vi "program seq..vi"(6 "IOList":T3, 7 "Cluster data":T5, 11 "Filepath":path=path "E:/My Project/2018-2019/Under development/Minda Ind. Switch -ID 144-145/Project/data/trail pro -12.txt") -> (0 "Error Out":errorcluster)   [LabVIEW 2015]
uses:
  Control PB/Active.ctl
  Control PB/deactive.ctl
  Control PB/output control.ctl
  Control PB/input control.ctl
  Control PB/timer.ctl
  Control PB/Remove list.ctl
  Control Button/Exit.ctl
  Control PB/Add_s.ctl
  Control PB/Delete_.ctl
  Control Button/Save.ctl
  Control PB/motor.ctl
  Control PB/Camera.ctl
  Control PB/Barcode.ctl
  Galobal variable_TI.vi
panel:
  out "Step List 4":string[](array[string])
  out "Step List 3":string[](array[string])
  in  "Barcode":T1
  in  "Camera":T2
  out "x <= y?":bool
  out "Cancel":bool
  out "Step List 2":string[](array[string])
  out "Pokayoka Result":cluster{"Sensor Name":string, "Boolean":bool}[](array[cluster])
  in  "Feed Back Channel":i32[](listbox)=[0]
  out "Input":bool[](array[boolean])
  out "Feature List (Out) 2":T4(array[cluster])
  out "error out 2":errorcluster
  in  "Control":bool
  out "Station No":string
  out "Model Name":string
  out "Model":string
  in  "Motor":T6
  in  "Feature List":i32(listbox) caption="Steps List"
  in  "Deletefeature list":T7
  in  "Add feature list":T8
  in  "Deactive":T9
  in  "Active":T10
  in  "Program step":i32(listbox)
  in  "Remove Step":T11
  in  "Wait Time":u32=100 caption="Timer(ms)" max=600000 step=1
  in  "Timer":T12
  in  "Save":T13
  in  "stop":T14
  in  "op Add":T15
  in  "Input Add":T16
  out "Step List":string[](array[string])
  out "output cluster":T17
  in  "Analog":bool
  in  "Analog Input":i32[](listbox)=[0]
  in  "Control Channel":i32[](listbox)=[7]
  in  "Steps":T18(array[cluster])
  in  "Program mode":string="Data"
  out "error out":errorcluster
  out "Feature List (Out)":T19(array[cluster])
  # "Program Sequence Window"
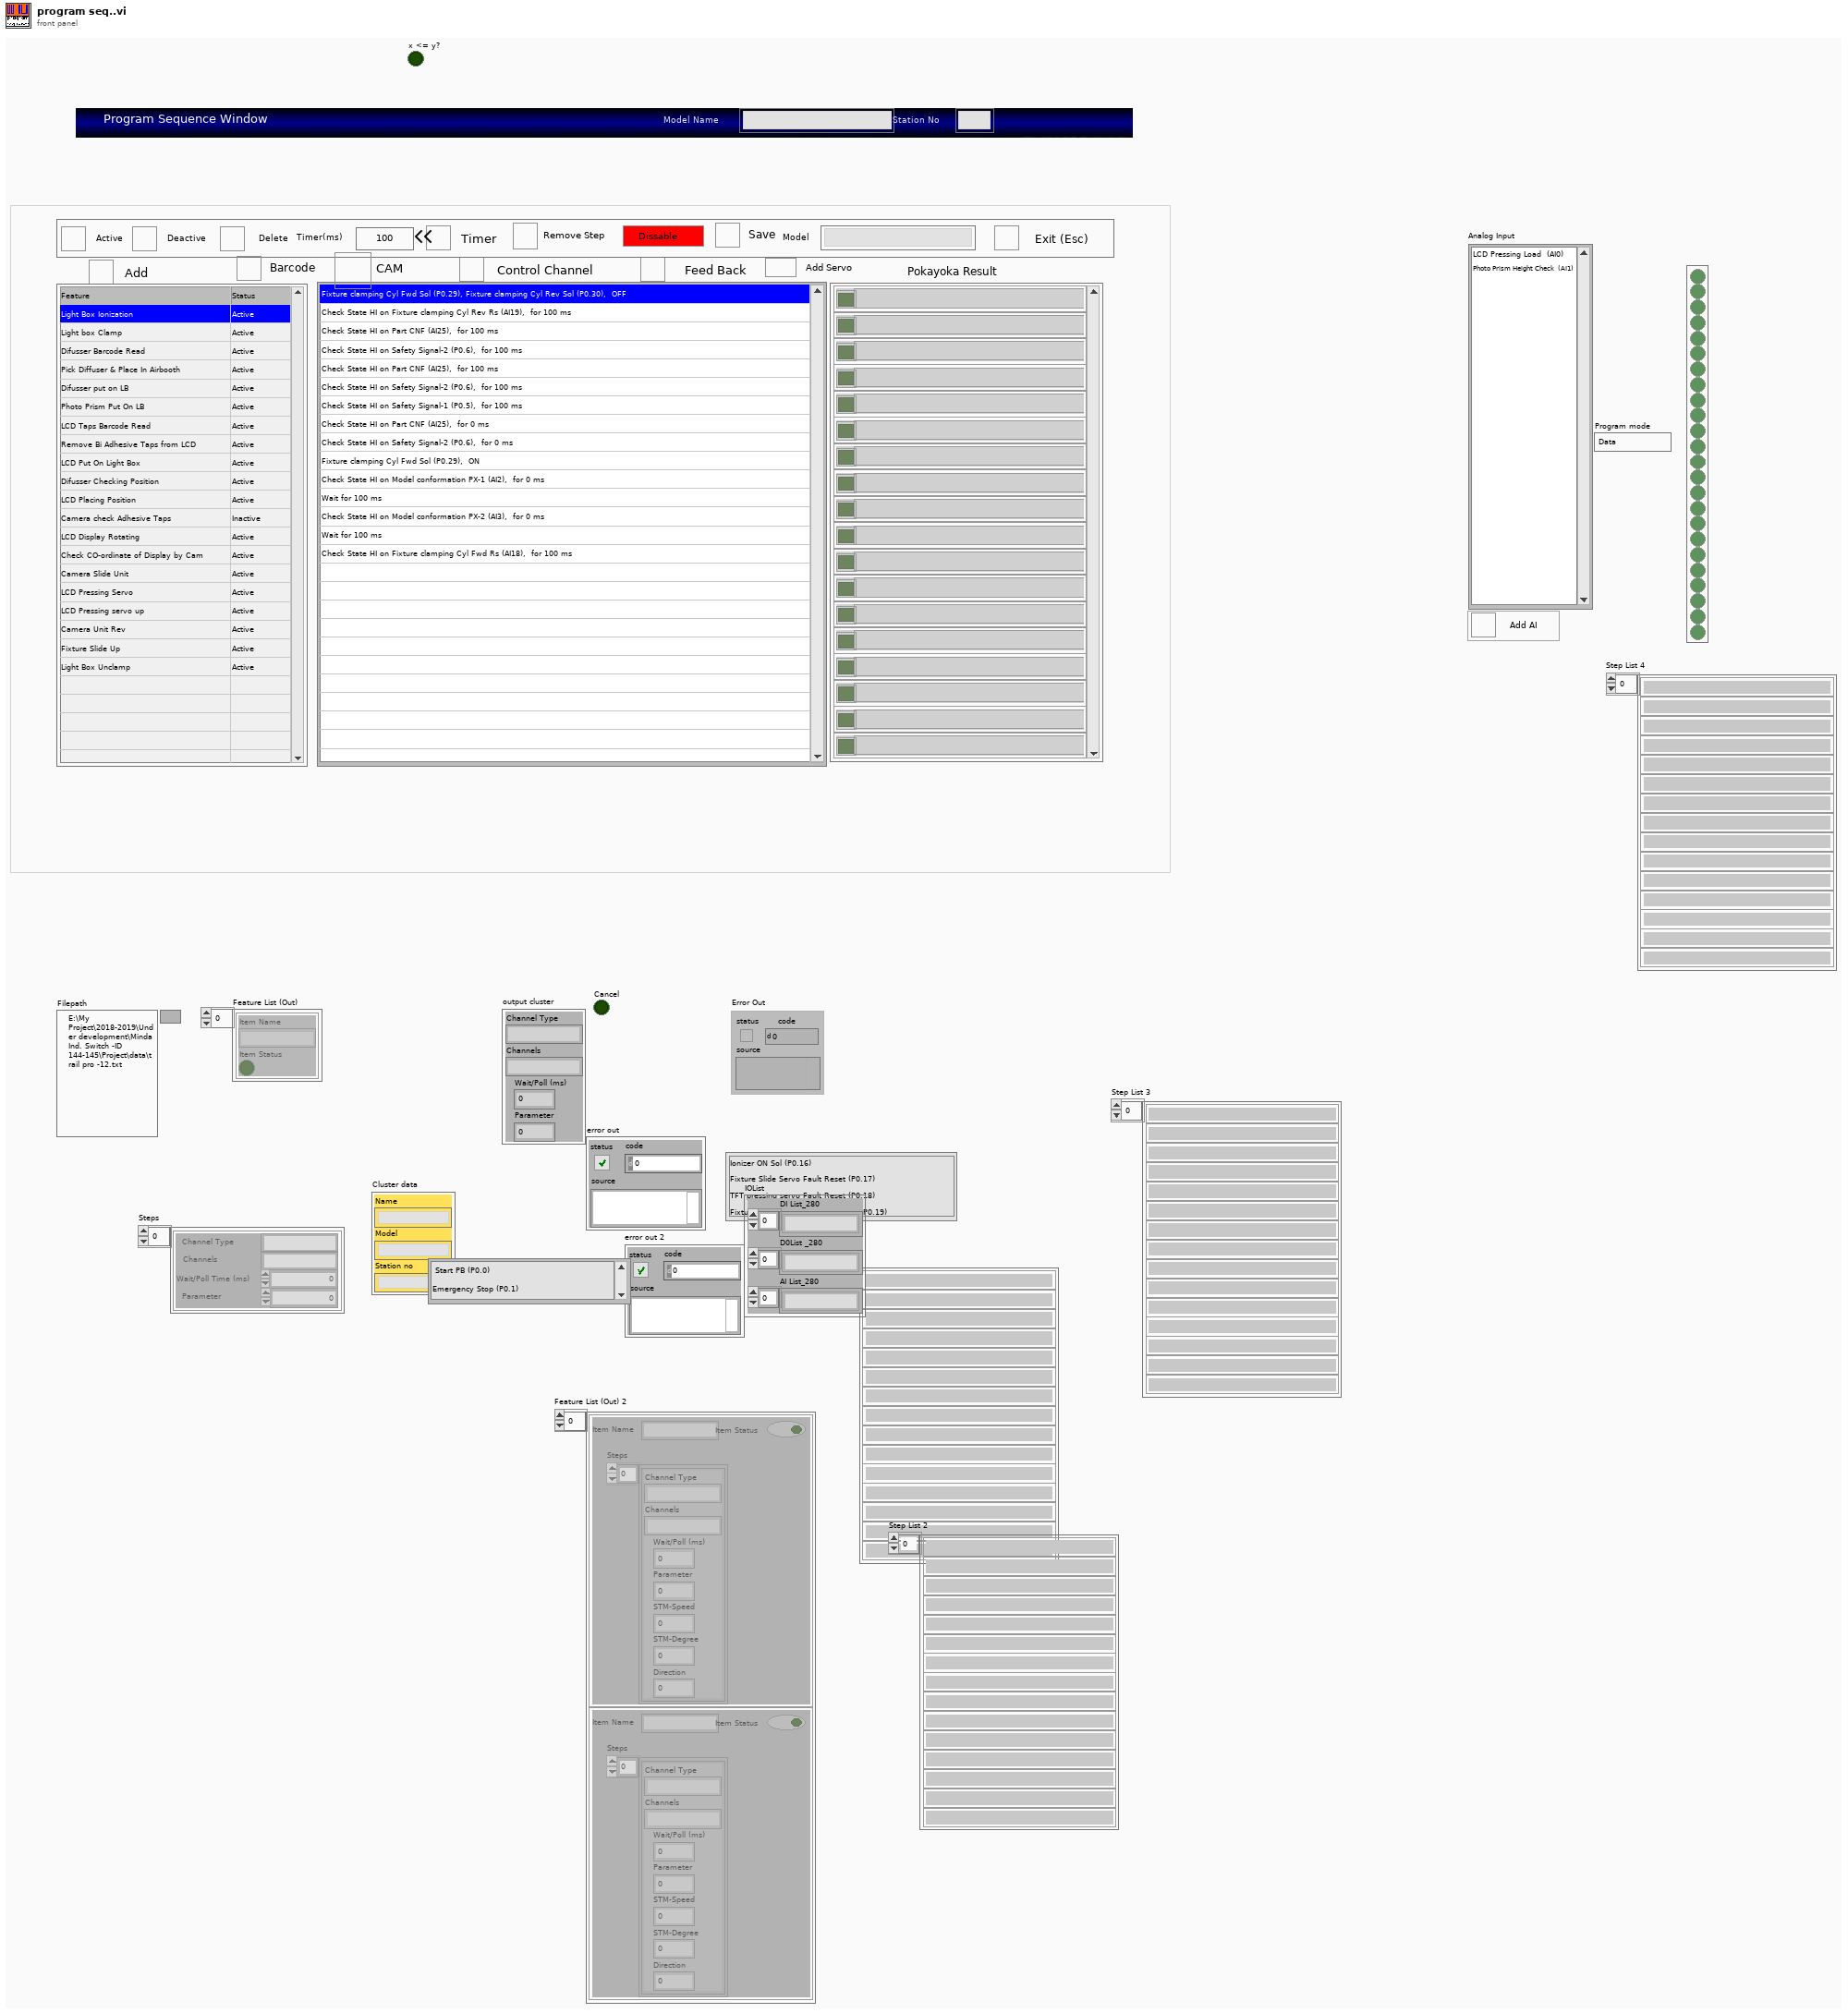
[diagram p1: front panel]
types:
  T1 = typedef "Barcode.ctl" = bool
  T2 = typedef "Camera.ctl" = bool
  T3 = cluster{"DI List_280":string[], "D0List _280":string[], "AI List_280":string[]}
  T4 = cluster{"Item Name":string, "Item Status":bool, "Steps":cluster{"Channel Type":string, "Channels":string, "Wait/Poll (ms)":u32, "Parameter":u8, "STM-Speed":i32, "STM-Degree":u32, "Direction":u8}[]}[]
  T5 = cluster{"Name":string, "Model":string, "Station no":string}
  T6 = typedef "motor.ctl" = bool
  T7 = typedef "Delete_.ctl" = bool
  T8 = typedef "Add_s.ctl" = bool
  T9 = typedef "deactive.ctl" = bool
  T10 = typedef "Active.ctl" = bool
  T11 = typedef "Remove list.ctl" = bool
  T12 = typedef "timer.ctl" = bool
  T13 = typedef "Save.ctl" = bool
  T14 = typedef "Exit.ctl" = bool
  T15 = typedef "output control.ctl" = bool
  T16 = typedef "input control.ctl" = bool
  T17 = cluster{"Channel Type":string, "Channels":string, "Wait/Poll (ms)":u32, "Parameter":u8}
  T18 = cluster{"Channel Type":string, "Channels":string, "Wait/Poll Time (ms)":u32, "Parameter":u8}[]
  T19 = cluster{"Item Name":string, "Item Status":bool}[]
  T20 = cluster{"Channel Type":string, "Channels":string, "Wait/Poll (ms)":u32, "Parameter":u8, "STM-Speed":i32, "STM-Degree":i32, "Direction":u8}
  T21 = cluster{"Item Name":string, "Item Status":bool, "Steps":cluster{"Channel Type":string, "Channels":string, "Wait/Poll (ms)":u32, "Parameter":u8, "STM-Speed":i32, "STM-Degree":u32, "Direction":u8}[]}
  T22 = cluster{"Channel Type":string, "Channels":string, "Wait/Poll (ms)":u32, "Parameter":u8, "STM-Speed":i32, "STM-Degree":u32, "Direction":u8}[]
  T23 = cluster{"Item Name":string, "Active":T10, "Steps":cluster{"Channel Type":string, "Channels":string, "Wait/Poll (ms)":u32, "Parameter":u8, "STM-Speed":i32, "STM-Degree":u32, "Direction":u8}[]}
  T24 = cluster{"Channel Type":string, "Channels":string, "Wait/Poll (ms)":u32, "Parameter":u8, "STM-Speed":i32, "STM-Degree":i32, "Direction":u8}[]
  T25 = cluster{"Feature name ":string, bool, cluster{"Channel Type":string, "Channels":string, "Wait/Poll (ms)":u32, "Parameter":u8, "STM-Speed":i32, "STM-Degree":i32, "Direction":u8}[]}
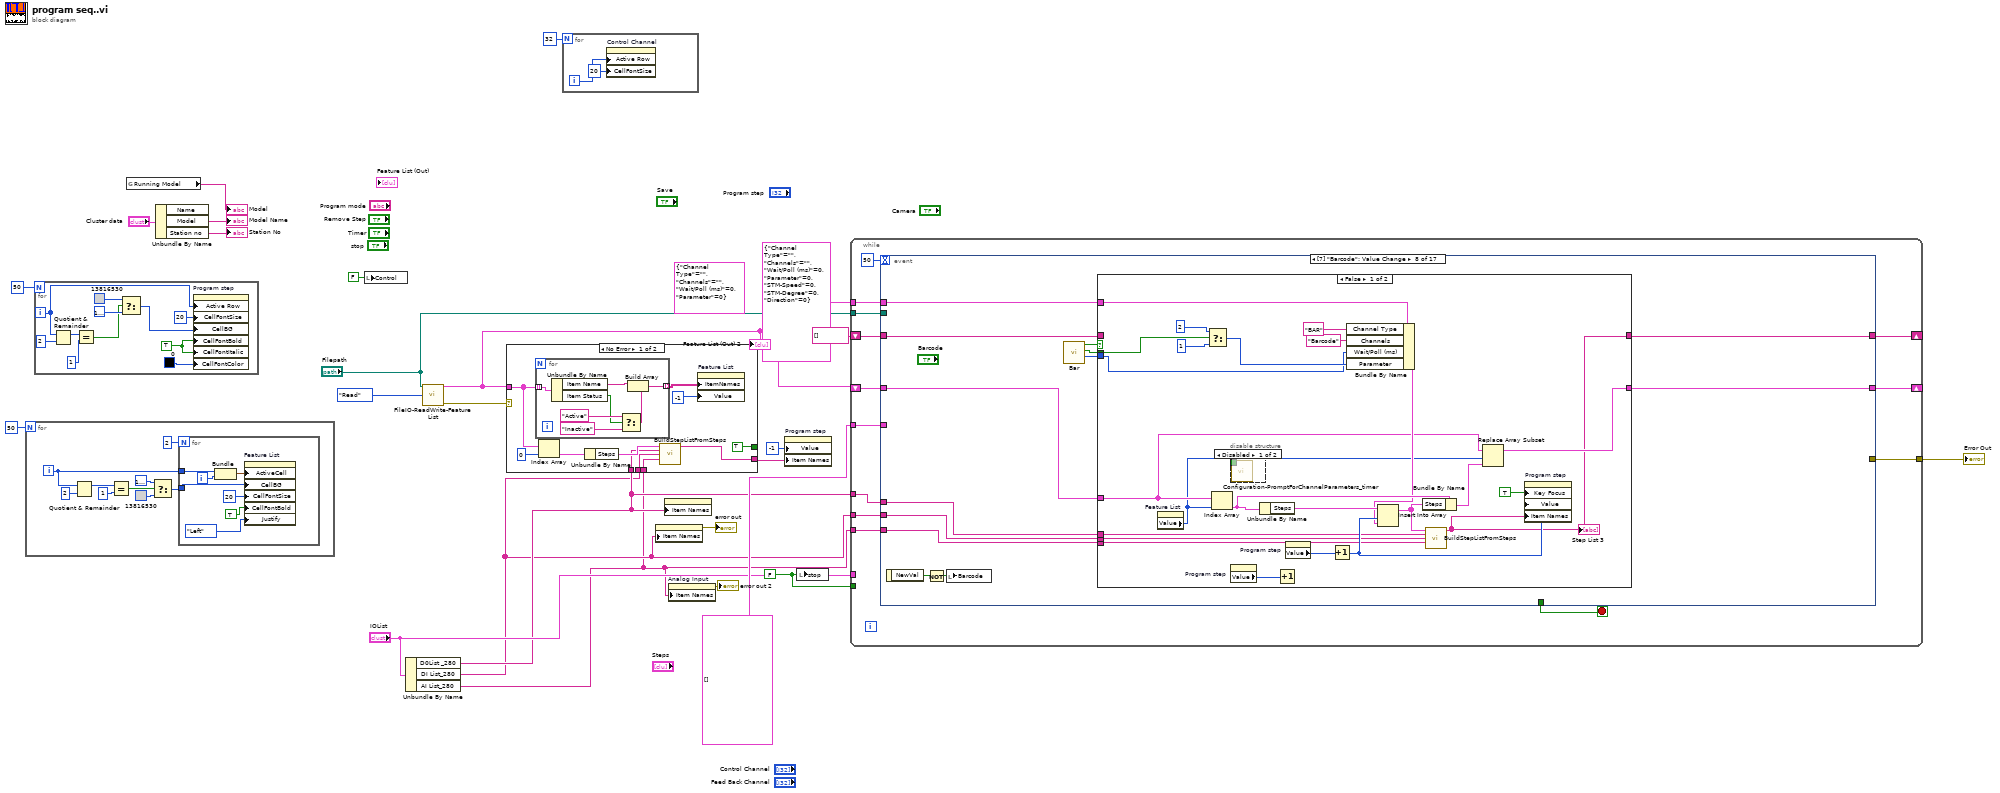
[diagram p0: block diagram]
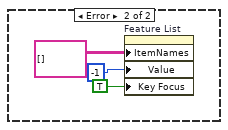
[diagram p2: hidden frame]
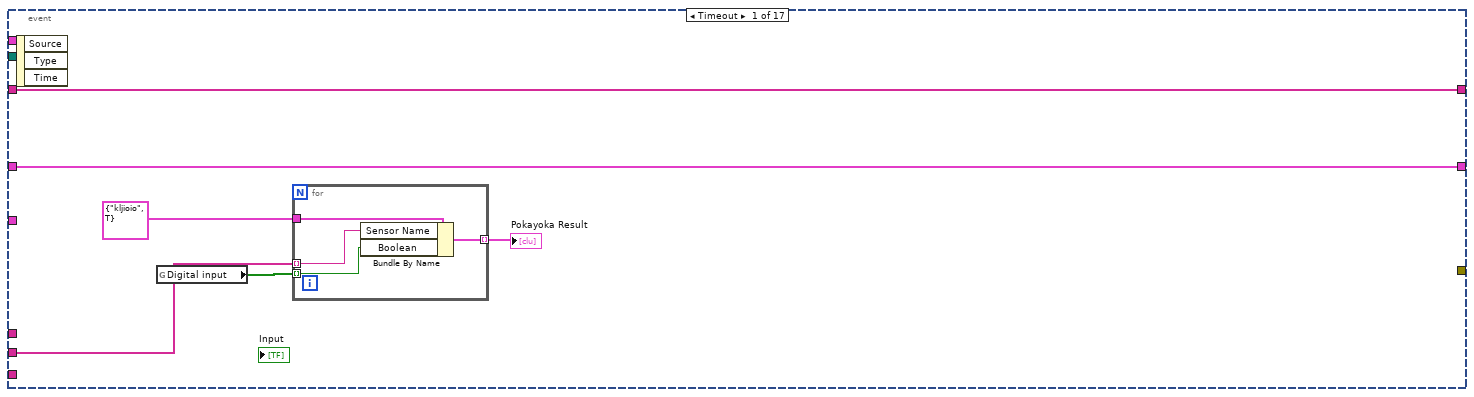
[diagram p3: hidden frame]
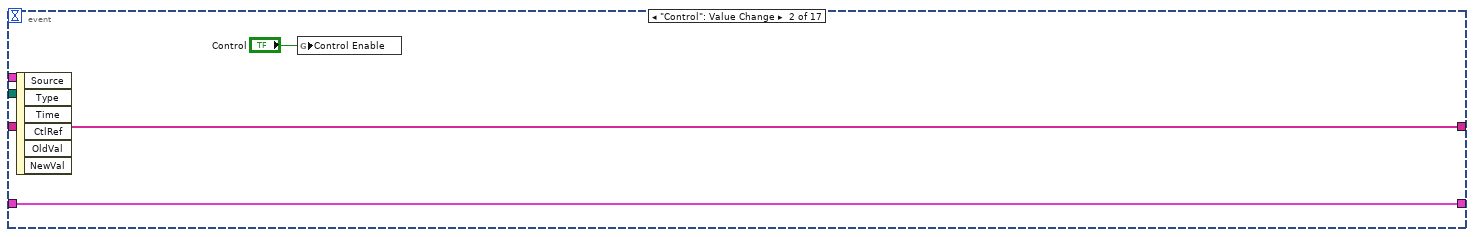
[diagram p4: hidden frame]
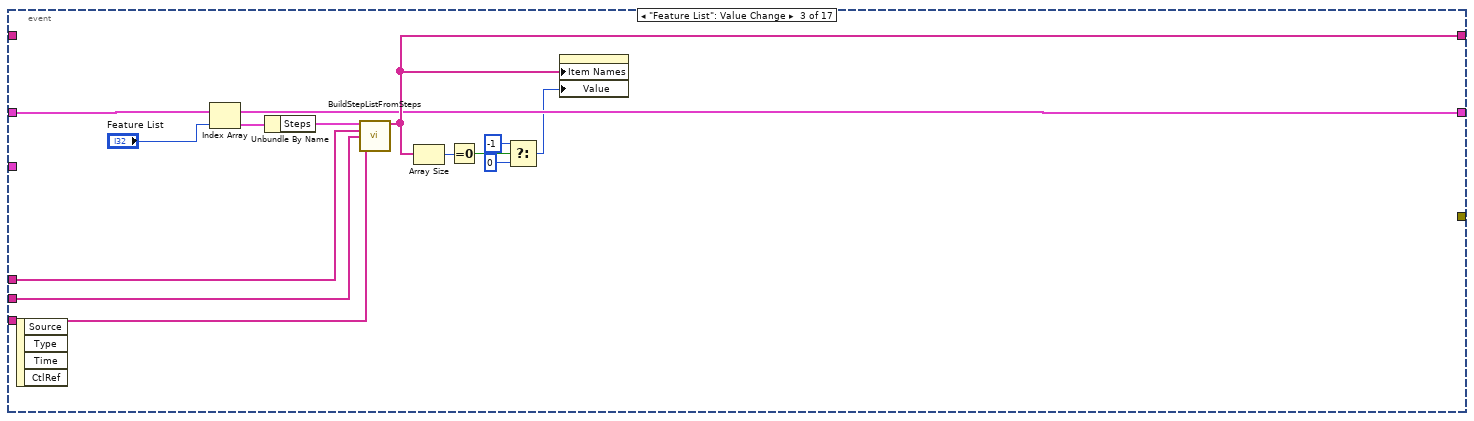
[diagram p5: hidden frame]
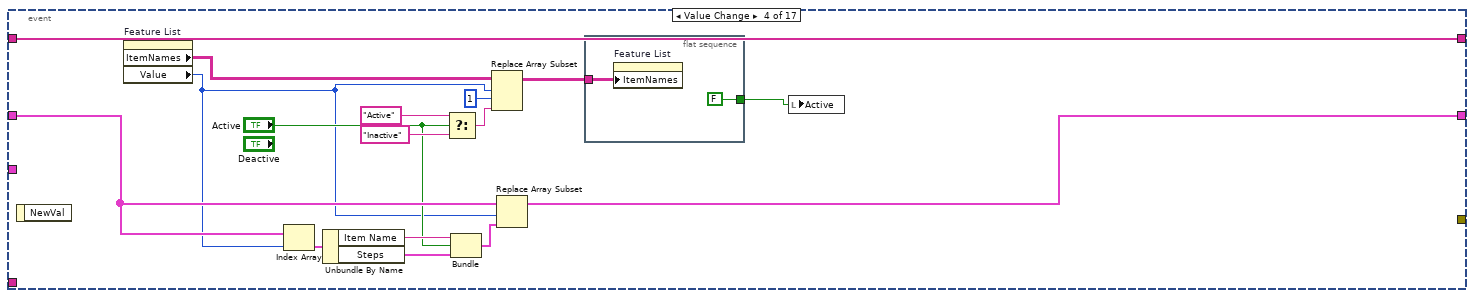
[diagram p6: hidden frame]
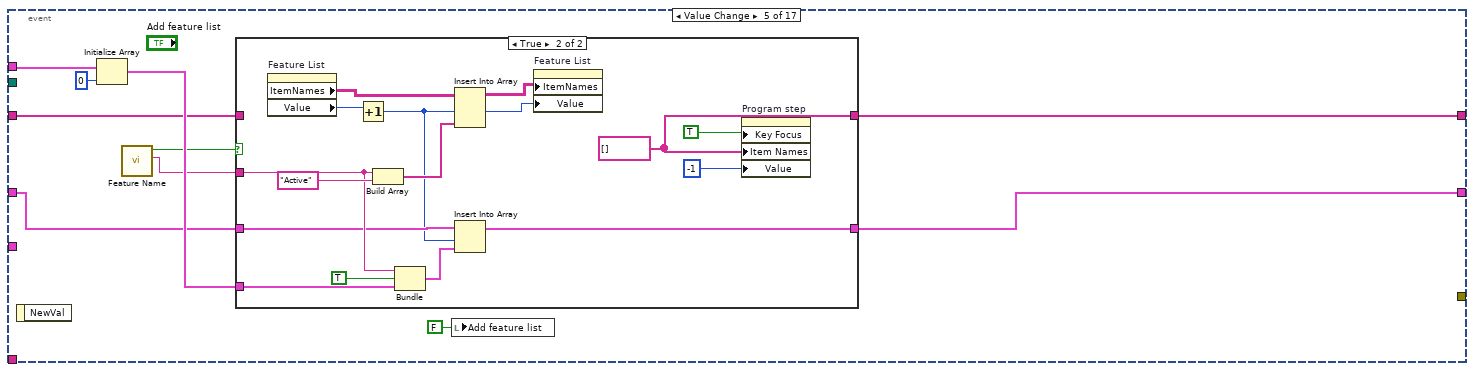
[diagram p7: hidden frame]
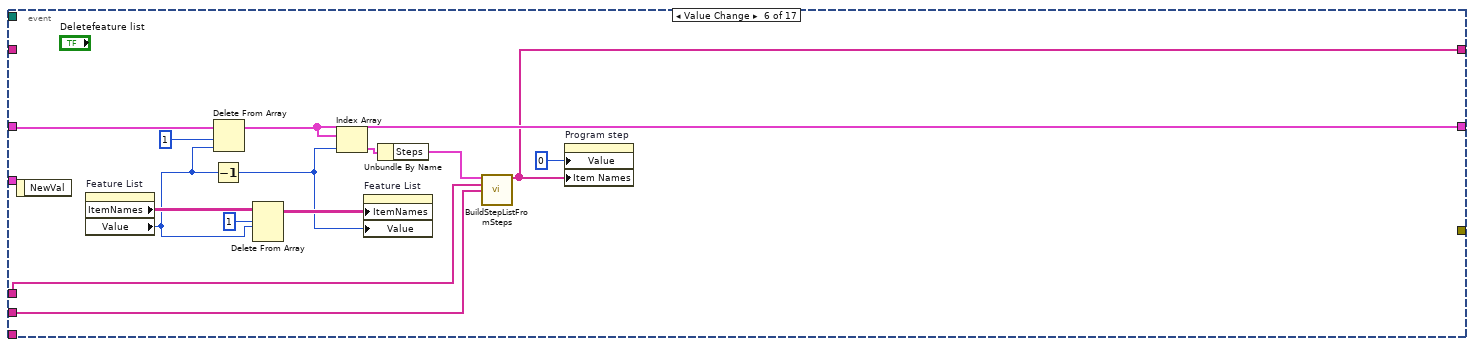
[diagram p9: hidden frame]
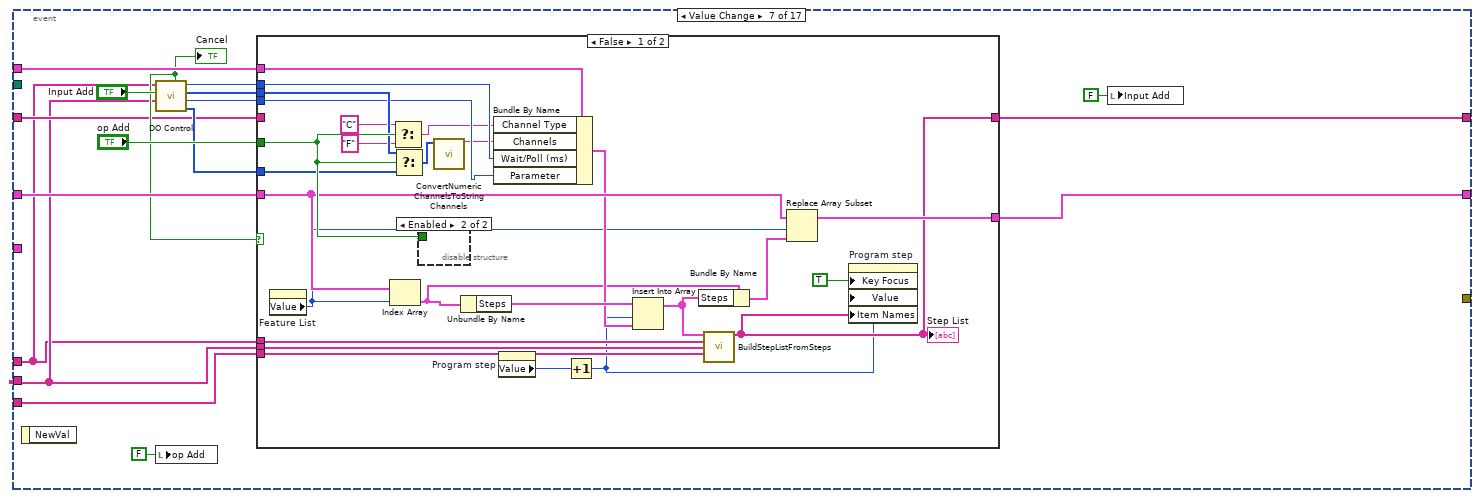
[diagram p10: hidden frame]
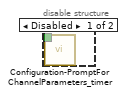
[diagram p11: hidden frame]
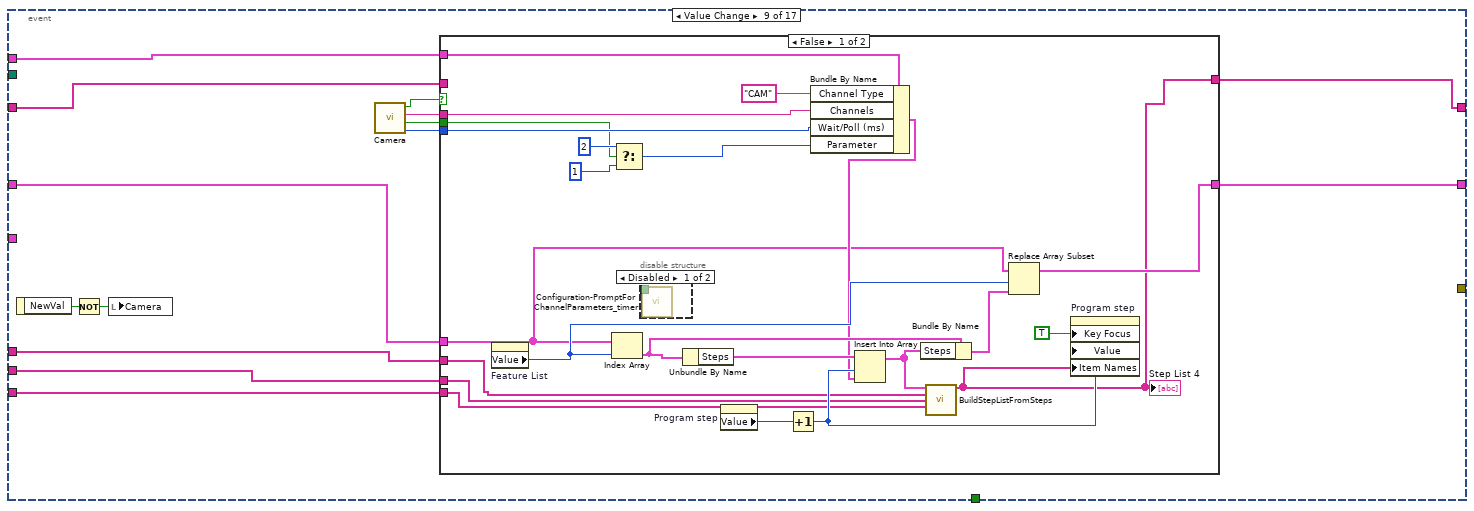
[diagram p15: hidden frame]
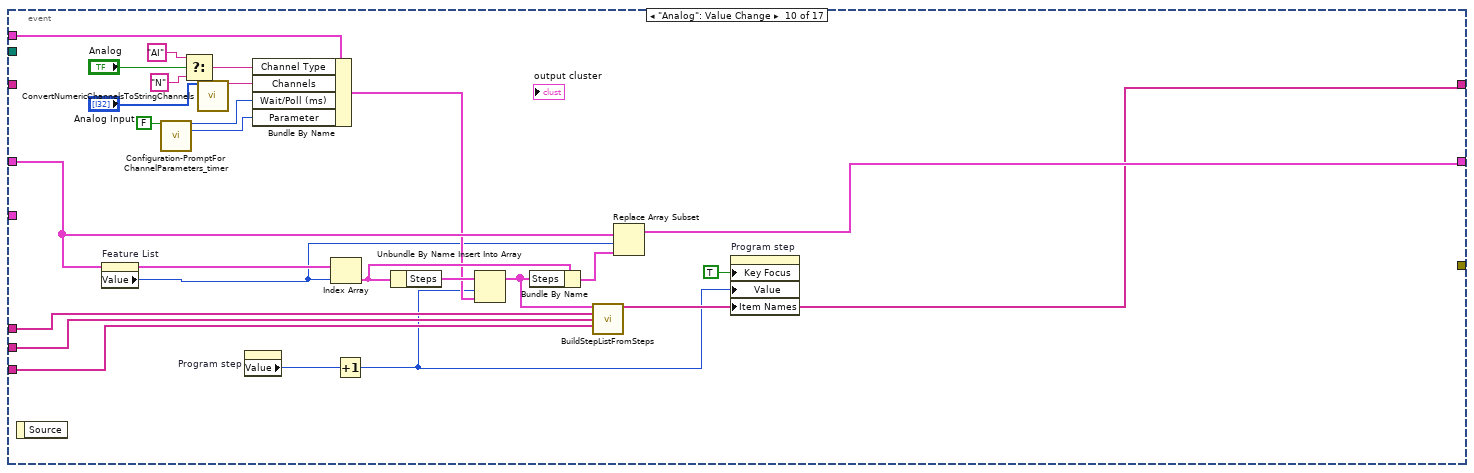
[diagram p18: hidden frame]
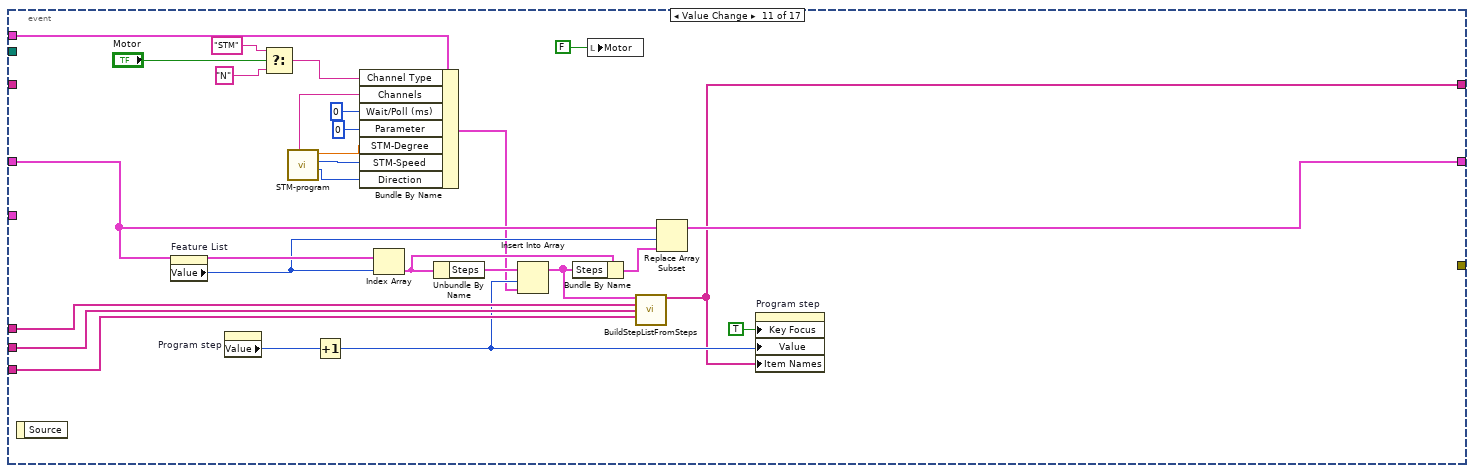
[diagram p19: hidden frame]
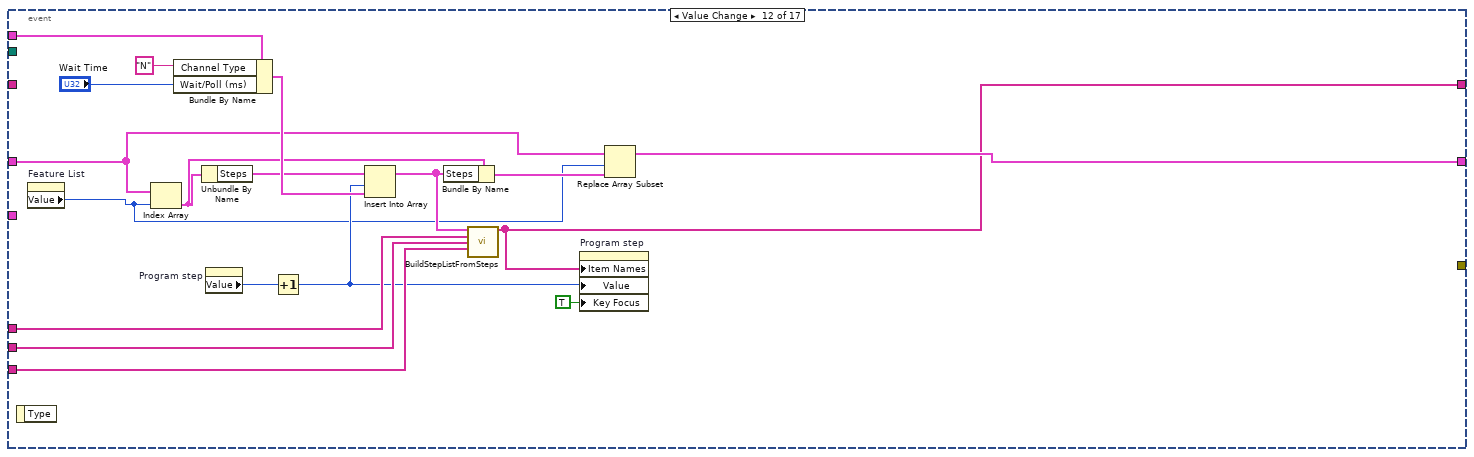
[diagram p20: hidden frame]
diagram:
  w9 = FALSE ("stop")
  (unwired) T17 {"Channel Type"="", "Channels"="", "Wait/Poll (ms)"=0, "Parameter"=0} ("Step")
  n1 = for {
    N: 50 -> [_]
    i -> [w33]
    n2 = Quotient & Remainder(x=w33, y=2) -> (x-y*floor(x/y)=w31:i32)  [unwired: 1 out]
    n3 = Equal?(x=w31, y=1) -> (x = y?=w29:bool)
    n4 = Select(t=u32 16777225 ("Color Box"), s=w29, f=u32 13816530 ("Color Box")) -> (s? t:f=w26:u32)
    n5 = for {
      N: 2 -> [_]
      tunnel: w33 -> [w41]
      tunnel: w26 -> [w38]
      i -> [w40]
      n6 = Bundle(w41, w40) -> (w39:cluster{i32, i32})  [unwired: 1 in]
      n7 = property on="Feature List" class="MCListbox (strict)"("ActiveCell"=w39, "CellBG"=w38, "CellFontSize"=u32 20 ("Active Cell:Cell Font:Size"), "CellFontBold"=TRUE ("Active Cell:Cell Font:Bold"), "Justify"=enum16{"Left", "Center", "Right"}."Left" ("Active Cell:Cell Justification")) -> ()  [unwired: 2 in, 2 out]
    }
  }
  n8 = for {
    N: 50 -> [_]
    i -> [w46]
    w43 = TRUE
    n9 = Quotient & Remainder(x=w46, y=2) -> (x-y*floor(x/y)=w49:i32)  [unwired: 1 out]
    n10 = Equal?(x=w49, y=1) -> (x = y?=w47:bool)
    n11 = Select(t=u32 13816530 ("Color Box"), s=w47, f=u32 16777226 ("Color Box")) -> (s? t:f=w44:u32)
    n12 = property on="Program step" class="LstBox (strict)"("Active Row"=w46, "CellFontSize"=u32 20 ("Active Row:Cell Font:Size"), "CellBG"=w44, "CellFontBold"=w43, "CellFontItalic"=w43, "CellFontColor"=u32 0 ("Color Box")) -> ()  [unwired: 2 in, 2 out]
  }
  n13 = global read "Galobal variable_TI.vi" "Running Model"() -> (→"Model":string)
  n14 = Unbundle By Name("Cluster data") -> ("Model"=→"Model Name":string, "Station no"=→"Station No":string)  [unwired: 1 out]
  n15 = local write "Control"(FALSE ("Control")) -> ()
  n16 = Unbundle By Name("IOList") -> ("D0List _280"=w5:string[], "DI List_280"=w4:string[], "AI List_280"=w3:string[])
  n17 = call "FileIO-ReadWrite-FeatureList.vi"("Filepath"="Filepath", "Read/Write"=enum16{"Read", "Write"}."Read") -> ("Feature List (Out)"=w16:T4, "Error Out"=w20:errorcluster)  [unwired: 12 in]
  "Feature List (Out) 2" <- w16
  n18 = case shown="No Error" w20 {
    tunnel: w16 -> [w63 _]
    tunnel: w5 -> [w59 _]
    tunnel: w4 -> [w58 _]
    tunnel: w3 -> [w57 _]
    tunnel: [w56 _] -> w19
    tunnel: [TRUE ("Key Focus") _] -> _
    frame No Error {
      n19 = for {
        tunnel: w63 -> [w70] mode=indexing
        tunnel: [w64] -> w54 mode=indexing
        n20 = Unbundle By Name(w70) -> ("Item Name"=w66:string, "Item Status"=w67:bool)
        n21 = Select(t="Active", s=w67, f="Inactive") -> (s? t:f=w65:string)
        n22 = Build Array(w66, w65) -> (w64:string[])
      }
      n23 = Index Array(array=w63, index=0) -> (element=w61:T21)
      n24 = Unbundle By Name(w61) -> ("Steps"=w60:T22)
      n25 = call "BuildStepListFromSteps.vi"("Steps"=w60, "Control Channels"=w59, "Feedback Channels"=w58, "AI"=w57) -> ("Step List"=w56:string[])  [unwired: 11 in]
      n26 = property on="Feature List" class="MCListbox (strict)"("ItemNames"=w54, "Value"=-1 ("Feautre list")) -> ()  [unwired: 2 in, 2 out]
    }
    frame Error {
      n27 = property on="Feature List" class="MCListbox (strict)"("ItemNames"=string[][] [] ("Item Names"), "Value"=-1 ("Feautre list"), "Key Focus"=TRUE) -> ()  [unwired: 2 in, 2 out]
    }
  }
  n28 = for {
    N: 32 -> [_]
    i -> [w75]
    n29 = property on="Control Channel" class="LstBox (strict)"("Active Row"=w75, "CellFontSize"=u32 20 ("Active Row:Cell Font:Size")) -> ()  [unwired: 2 in, 2 out]
  }
  n30 = property on="Feed Back Channel" class="LstBox (strict)"("Item Names"=w4) -> (error out=→"error out":errorcluster)  [unwired: 2 in, 1 out]
  n31 = property on="Control Channel" class="LstBox (strict)"("Item Names"=w5) -> ()  [unwired: 2 in, 2 out]
  n32 = property on="Analog Input" class="LstBox (strict)"("Item Names"=w3) -> (error out=→"error out 2":errorcluster)  [unwired: 2 in, 1 out]
  n33 = property on="Program step" class="LstBox (strict)"("Value"=-1 ("Step feautre list"), "Item Names"=w19) -> ()  [unwired: 2 in, 2 out]
  n34 = local write "stop"(w9) -> ()
  n35 = while {
    shift-right: [w86] -> _
    shift-left: w16 -> [w77]
    tunnel: T20 {"Channel Type"="", "Channels"="", "Wait/Poll (ms)"=0, "Parameter"=0, "STM-Speed"=0, "STM-Degree"=0, "Direction"=0} ("Step") -> [w87]
    shift-right: [w85] -> _
    shift-left: string[] [] ("Step List") -> [w84]
    tunnel: w5 -> [w83]
    tunnel: w4 -> [w82]
    tunnel: [w81] -> w23
    tunnel: w3 -> [w80]
    tunnel: T4 [] ("Feature List (Out) 2") -> [w79]
    tunnel: "Filepath" -> [w78]
    tunnel: w9 -> [_]
    tunnel: "IOList" -> [_]
    stop <- w88 stop-if-true
    n36 = event shown="[7] \"Barcode\": Value Change" {
      selector: _ -> [_ _ _ _ _ _ _ _ _ _ _ _ _ _ _ _ _]
      dyn-events: _ -> [_ _ _ _ _ _ _ _ _ _ _ _ _ _ _ _ _]
      timeout: 50 -> [_ _ _ _ _ _ _ _ _ _ _ _ _ _ _ _ _]
      tunnel: [_ _ _ _ _ _ _ _ _ _ _ _ _ _ TRUE ("stop") _ TRUE ("Discard?")] -> w88
      tunnel: w77 -> [w94 w100 w105 w122 w139 w171 w187 w227 w269 w309 w339 w360 w382 w391 w451 w473 w550]
      tunnel: w87 -> [_ _ _ _ w142 _ w190 w232 w273 w316 w344 w369 _ _ _ w474 _]
      tunnel: [w94 w100 w105 w120 w138 w170 w188 w226 w268 w304 w331 w359 w381 w393 w451 w469 w550] -> w86
      tunnel: [w93 w101 w108 w119 w135 w165 w186 w225 w267 w303 w330 w356 w376 w408 w450 w468 w551] -> w85
      tunnel: w84 -> [w93 w101 _ w119 w134 _ w177 w220 w263 _ _ _ _ _ w450 w467 w551]
      tunnel: w83 -> [_ _ w107 _ _ w167 w175 w228 w270 w306 w336 w358 w378 w410 _ w470 _]
      tunnel: w82 -> [w92 _ w106 _ _ w166 w176 w229 w271 w307 w335 w357 w377 w409 _ w471 _]
      tunnel: [_ _ _ _ _ _ _ _ _ _ _ _ _ w401 _ _ _] -> w81
      tunnel: w80 -> [_ _ w104 _ _ _ w185 w230 w272 w308 w334 w355 _ w402 _ w472 _]
      tunnel: w79 -> [_ _ _ _ _ _ _ _ _ _ _ _ _ w407 _ _ _]
      tunnel: w78 -> [_ _ _ _ _ _ _ _ _ _ _ _ _ w392 _ _ _]
      event Timeout {
        n37 = event-data() -> ()  [unwired: 1 in, 3 out]
        n38 = global read "Galobal variable_TI.vi" "Digital input"() -> (w89:bool[])
        n39 = for {
          tunnel: w92 -> [w97] mode=indexing
          tunnel: cluster{"Sensor Name":string, "Boolean":bool} {"Sensor Name"="kljioio", "Boolean"=TRUE} ("Cluster") -> [w98]
          tunnel: [w96] -> w90 mode=indexing
          tunnel: w89 -> [w95] mode=indexing
          n40 = Bundle By Name(cluster=w98, "Sensor Name"=w97, "Boolean"=w95) -> (w96:cluster{"Sensor Name":string, "Boolean":bool})
        }
        "Pokayoka Result" <- w90
      }
      event "Control": Value Change {
        n41 = event-data() -> ()  [unwired: 1 in, 6 out]
        n42 = global write "Galobal variable_TI.vi" "Control Enable"("Control") -> ()
      }
      event "Feature List": Value Change {
        n43 = event-data() -> ()  [unwired: 1 in, 4 out]
        n44 = Index Array(array=w105, index="Feature List") -> (element=w114:T21)
        n45 = Unbundle By Name(w114) -> ("Steps"=w113:T22)
        n46 = call "BuildStepListFromSteps.vi"("Steps"=w113, "Control Channels"=w107, "Feedback Channels"=w106, "AI"=w104) -> ("Step List"=w108:string[])  [unwired: 11 in]
        n47 = Array Size(array=w108) -> (size(s)=w110:i32)
        n48 = Equal To 0?(x=w110) -> (x = 0?=w112:bool)
        n49 = Select(t=-1 ("Step List"), s=w112, f=0 ("Step List")) -> (s? t:f=w103:i32)
        n50 = property on="Program step" class="LstBox (strict)"("Item Names"=w108, "Value"=w103) -> ()  [unwired: 2 in, 2 out]
      }
      event Value Change {
        n51 = event-data() -> ()  [unwired: 1 in, 1 out]
        n52 = property on="Feature List" class="MCListbox (strict)"() -> ("ItemNames"=w118:string[][], "Value"=w116:i32)  [unwired: 2 in, 2 out]
        n53 = Index Array(array=w122, index=w116) -> (element=w128:T21)
        n54 = Unbundle By Name(w128) -> ("Item Name"=w129:string, "Steps"=w130:T22)
        n55 = Select(t="Active", s="Active", f="Inactive" ("element")) -> (s? t:f=w125:string)
        n56 = Bundle("Item Name"=w129, "Active"="Active", "Steps"=w130) -> (w127:T23)  [unwired: 1 in]
        n57 = Replace Array Subset(array=w118, new element=w125, index (row)=w116, index (col)=1 ("disabled index (col)")) -> (w117:string[][])
        n58 = Replace Array Subset(array=w122, new element=w127, index=w116) -> (w120:T4)
        n59 = flat-sequence {
          tunnel: w117 -> [w132]
          tunnel: [T10 FALSE ("Active")] -> w115
          frame #0 {
            n60 = property on="Feature List" class="MCListbox (strict)"("ItemNames"=w132) -> ()  [unwired: 2 in, 2 out]
          }
        }
        n61 = local write "Active"(w115) -> ()
      }
      event Value Change {
        n62 = event-data() -> ()  [unwired: 1 in, 1 out]
        n63 = Initialize Array(w142, 0 ("dimension size")) -> (w140:T24)
        n64 = call "Feature Name.vi"() -> ("Feature name"=w136:string, "Out"=w137:bool)  [unwired: 10 in]
        n65 = case shown="True" w137 {
          tunnel: w140 -> [_ w158]
          tunnel: w139 -> [w144 w153]
          tunnel: [w144 w155] -> w138
          tunnel: w136 -> [_ w154]
          tunnel: [w143 w151] -> w135
          tunnel: w134 -> [w143 _]
          frame False {
          }
          frame True {
            w151 = string[] [] ("Item Names")
            n66 = property on="Feature List" class="MCListbox (strict)"() -> ("ItemNames"=w148:string[][], "Value"=w145:i32)  [unwired: 2 in, 2 out]
            n67 = Increment(x=w145) -> (x+1=w146:i32)
            n68 = Build Array(w154, "Active") -> (w149:string[])
            n69 = Bundle("Feature name"=w154, TRUE, w158) -> (w156:T25)  [unwired: 1 in]
            n70 = Insert Into Array(array=w148, index (row)=w146, new element=w149) -> (w147:string[][])  [unwired: 1 in]
            n71 = Insert Into Array(array=w153, index=w146, new element=w156) -> (w155:T4)
            n72 = property on="Feature List" class="MCListbox (strict)"("ItemNames"=w147, "Value"=w146) -> ()  [unwired: 2 in, 2 out]
            n73 = property on="Program step" class="LstBox (strict)"("Key Focus"=TRUE, "Item Names"=w151, "Value"=-1 ("Step feautre list")) -> ()  [unwired: 2 in, 2 out]
          }
        }
        n74 = local write "Add feature list"(FALSE ("Add feature list")) -> ()
      }
      event Value Change {
        n75 = event-data() -> ()  [unwired: 1 in, 1 out]
        n76 = property on="Feature List" class="MCListbox (strict)"() -> ("ItemNames"=w163:string[][], "Value"=w162:i32)  [unwired: 2 in, 2 out]
        n77 = Decrement(x=w162) -> (x-1=w160:i32)
        n78 = Delete From Array(array=w171, length=1, index=w162) -> (array with subset deleted=w170:T4)  [unwired: 1 out]
        n79 = Delete From Array(array=w163, length=1, index (row)=w162) -> (array with subset deleted=w161:string[][])  [unwired: 1 in, 1 out]
        n80 = Index Array(array=w170, index=w160) -> (element=w169:T21)
        n81 = property on="Feature List" class="MCListbox (strict)"("ItemNames"=w161, "Value"=w160) -> ()  [unwired: 2 in, 2 out]
        n82 = Unbundle By Name(w169) -> ("Steps"=w168:T22)
        n83 = call "BuildStepListFromSteps.vi"("Steps"=w168, "Control Channels"=w167, "Feedback Channels"=w166) -> ("Step List"=w165:string[])  [unwired: 12 in]
        n84 = property on="Program step" class="LstBox (strict)"("Value"=0 ("Step feautre list"), "Item Names"=w165) -> ()  [unwired: 2 in, 2 out]
      }
      event Value Change {
        n85 = event-data() -> ()  [unwired: 1 in, 1 out]
        n86 = call "DO Control.vi"("DI List_280"=w176, "s"="Input Add", "Control"=w175) -> ("Feedback"=w180:i32[], "Parameter (Out)"=w182:u8, "Control Channel"=w184:i32[], "Poll Time (Out)"=w183:u32, "Cancel"=w178:bool)  [unwired: 3 in, 1 out]
        "Cancel" <- w178
        n87 = local write "op Add"(T15 FALSE ("op Add")) -> ()
        n88 = case shown="False" w178 {
          tunnel: w190 -> [w216 _]
          tunnel: "op Add" -> [w215 _]
          tunnel: [w214 w219] -> w188
          tunnel: w187 -> [w213 w219]
          tunnel: w175 -> [w212 _]
          tunnel: w176 -> [w211 _]
          tunnel: [w210 w218] -> w186
          tunnel: w185 -> [w209 _]
          tunnel: w184 -> [w208 _]
          tunnel: w183 -> [w207 _]
          tunnel: w182 -> [w206 _]
          tunnel: w180 -> [w205 _]
          tunnel: w177 -> [_ w218]
          frame False {
            n89 = property on="Feature List" class="MCListbox (strict)"() -> ("Value"=w191:i32)  [unwired: 2 in, 2 out]
            n90 = Index Array(array=w213, index=w191) -> (element=w197:T21)
            n91 = Select(t="C", s=w215, f="F") -> (s? t:f=w202:string)
            n92 = Select(t=w208, s=w215, f=w205) -> (s? t:f=w201:i32[])
            n93 = disable-structure shown="Enabled" {
              disable-tunnel: w215 -> [w217 _]
              frame Disabled {
                n94 = call "Configuration-PromptForChannelParameters_timer.vi"("Control/Feedback\n(Default: False = Feedback)"=w217) -> ()  [unwired: 13 in, 2 out]
              }
              frame Enabled {
              }
            }
            n95 = call "ConvertNumericChannelsToStringChannels.vi"("Channels (In)"=w201) -> ("Channels (A:B:C:D...) (Out)"=w200:string)  [unwired: 14 in]
            n96 = Unbundle By Name(w197) -> ("Steps"=w199:T22)
            n97 = Bundle By Name(cluster=w216, "Channel Type"=w202, "Channels"=w200, "Wait/Poll (ms)"=w207, "Parameter"=w206) -> (w198:T20)
            n98 = property on="Program step" class="LstBox (strict)"() -> ("Value"=w192:i32)  [unwired: 2 in, 2 out]
            n99 = Increment(x=w192) -> (x+1=w193:i32)
            n100 = Insert Into Array "Insert Into Array"(array=w199, index=w193, new element=w198) -> (w195:T22)
            n101 = Bundle By Name(cluster=w197, "Steps"=w195) -> (w196:T21)
            n102 = call "BuildStepListFromSteps.vi"("Steps"=w195, "Control Channels"=w212, "Feedback Channels"=w211, "AI"=w209) -> ("Step List"=w210:string[])  [unwired: 11 in]
            "Step List" <- w210
            n103 = Replace Array Subset(array=w213, new element=w196, index=w191) -> (w214:T4)
            n104 = property on="Program step" class="LstBox (strict)"("Key Focus"=TRUE, "Value"=w193, "Item Names"=w210) -> ()  [unwired: 2 in, 2 out]
          }
          frame True {
          }
        }
        n105 = local write "Input Add"(T16 FALSE ("Input Add")) -> ()
      }
      event Value Change {
        n106 = event-data() -> ("NewVal"=w223:T1)  [unwired: 1 in]
        n107 = Not(x=w223) -> (.not. x?=w222:T1)
        n108 = local write "Barcode"(w222) -> ()
        n109 = call "Bar.vi"() -> ("Time Out Value"=w224:u8, "Barcode Scane"=w231:bool, "Out"=w221:bool)  [unwired: 9 in]
        n110 = case shown="False" w221 {
          tunnel: w232 -> [w256 _]
          tunnel: w231 -> [w253 _]
          tunnel: w230 -> [w240 _]
          tunnel: w229 -> [w239 _]
          tunnel: w228 -> [w238 _]
          tunnel: w227 -> [w237 w258]
          tunnel: [w236 w258] -> w226
          tunnel: [w235 w259] -> w225
          tunnel: w224 -> [w234 _]
          tunnel: w220 -> [_ w259]
          frame False {
            n111 = property on="Feature List" class="MCListbox (strict)"() -> ("Value"=w233:i32)  [unwired: 2 in, 2 out]
            n112 = Select(t=2, s=w253, f=1) -> (s? t:f=w250:i32)
            n113 = Index Array(array=w237, index=w233) -> (element=w248:T21)
            n114 = disable-structure shown="Disabled" {
              disable-tunnel: _ -> [w257 _]
              frame Disabled {
                n115 = call "Configuration-PromptForChannelParameters_timer.vi"("Control/Feedback\n(Default: False = Feedback)"=w257) -> ()  [unwired: 13 in, 2 out]
              }
              frame Enabled {
              }
            }
            n116 = property on="Program step" class="LstBox (strict)"() -> ("Value"=w242:i32)  [unwired: 2 in, 2 out]
            n117 = Unbundle By Name(w248) -> ("Steps"=w249:T22)
            n118 = Increment(x=w242) -> ()  [unwired: 1 out]
            n119 = property on="Program step" class="LstBox (strict)"() -> ("Value"=w243:i32)  [unwired: 2 in, 2 out]
            n120 = Increment(x=w243) -> (x+1=w244:i32)
            n121 = Bundle By Name(cluster=w256, "Channel Type"="BAR", "Channels"="Barcode", "Wait/Poll (ms)"=w234, "Parameter"=w250) -> (w241:T20)
            n122 = Insert Into Array "Insert Into Array"(array=w249, index=w244, new element=w241) -> (w246:T22)
            n123 = Bundle By Name(cluster=w248, "Steps"=w246) -> (w247:T21)
            n124 = call "BuildStepListFromSteps.vi"("Steps"=w246, "Control Channels"=w238, "Feedback Channels"=w239, "AI"=w240) -> ("Step List"=w235:string[])  [unwired: 11 in]
            "Step List 3" <- w235
            n125 = Replace Array Subset(array=w237, new element=w247, index=w233) -> (w236:T4)
            n126 = property on="Program step" class="LstBox (strict)"("Key Focus"=TRUE, "Value"=w244, "Item Names"=w235) -> ()  [unwired: 2 in, 2 out]
          }
          frame True {
          }
        }
      }
      event Value Change {
        n127 = event-data() -> ("NewVal"=w260:T2)  [unwired: 1 in]
        n128 = Not(x=w260) -> (.not. x?=w261:T2)
        n129 = local write "Camera"(w261) -> ()
        n130 = call "Camera.vi"() -> ("Time Out (ms) 2"=w265:u8, "Camera 2"=w264:bool, "Feature name"=w266:string, "Out"=w262:bool)  [unwired: 8 in]
        n131 = case shown="False" w262 {
          tunnel: w273 -> [w283 _]
          tunnel: w272 -> [w282 _]
          tunnel: w271 -> [w281 _]
          tunnel: w270 -> [w280 _]
          tunnel: w269 -> [w279 w298]
          tunnel: [w278 w298] -> w268
          tunnel: [w277 w299] -> w267
          tunnel: w266 -> [w276 _]
          tunnel: w265 -> [w275 _]
          tunnel: w264 -> [w274 _]
          tunnel: w263 -> [_ w299]
          frame False {
            n132 = property on="Feature List" class="MCListbox (strict)"() -> ("Value"=w285:i32)  [unwired: 2 in, 2 out]
            n133 = Index Array(array=w279, index=w285) -> (element=w291:T21)
            n134 = Select(t=2, s=w274, f=1) -> (s? t:f=w293:i32)
            n135 = disable-structure shown="Disabled" {
              disable-tunnel: _ -> [w297 _]
              frame Disabled {
                n136 = call "Configuration-PromptForChannelParameters_timer.vi"("Control/Feedback\n(Default: False = Feedback)"=w297) -> ()  [unwired: 13 in, 2 out]
              }
              frame Enabled {
              }
            }
            n137 = Unbundle By Name(w291) -> ("Steps"=w292:T22)
            n138 = property on="Program step" class="LstBox (strict)"() -> ("Value"=w286:i32)  [unwired: 2 in, 2 out]
            n139 = Increment(x=w286) -> (x+1=w287:i32)
            n140 = Bundle By Name(cluster=w283, "Channel Type"="CAM", "Channels"=w276, "Wait/Poll (ms)"=w275, "Parameter"=w293) -> (w284:T20)
            n141 = Insert Into Array "Insert Into Array"(array=w292, index=w287, new element=w284) -> (w289:T22)
            n142 = Bundle By Name(cluster=w291, "Steps"=w289) -> (w290:T21)
            n143 = call "BuildStepListFromSteps.vi"("Steps"=w289, "Control Channels"=w280, "Feedback Channels"=w281, "AI"=w282) -> ("Step List"=w277:string[])  [unwired: 11 in]
            "Step List 4" <- w277
            n144 = Replace Array Subset(array=w279, new element=w290, index=w285) -> (w278:T4)
            n145 = property on="Program step" class="LstBox (strict)"("Key Focus"=TRUE, "Value"=w287, "Item Names"=w277) -> ()  [unwired: 2 in, 2 out]
          }
          frame True {
          }
        }
      }
      event "Analog": Value Change {
        n146 = event-data() -> ()  [unwired: 1 in, 1 out]
        n147 = property on="Feature List" class="MCListbox (strict)"() -> ("Value"=w300:i32)  [unwired: 2 in, 2 out]
        n148 = call "Configuration-PromptForChannelParameters_timer.vi"("Control/Feedback\n(Default: False = Feedback)"=FALSE ("Control/Feedback\n(Default: False = Feedback)")) -> ("Poll Time (Out)"=w320:u32, "Parameter (Out)"=w319:u8)  [unwired: 13 in]
        n149 = Select(t="AI", s="Analog", f="N") -> (s? t:f=w322:string)
        n150 = call "ConvertNumericChannelsToStringChannels.vi"("Channels (In)"="Analog Input") -> ("Channels (A:B:C:D...) (Out)"=w321:string)  [unwired: 14 in]
        n151 = property on="Program step" class="LstBox (strict)"() -> ("Value"=w310:i32)  [unwired: 2 in, 2 out]
        n152 = Bundle By Name(cluster=w316, "Channel Type"=w322, "Channels"=w321, "Wait/Poll (ms)"=w320, "Parameter"=w319) -> (w305:T20)
        n153 = Index Array(array=w309, index=w300) -> (element=w314:T21)
        n154 = Increment(x=w310) -> (x+1=w301:i32)
        n155 = Unbundle By Name(w314) -> ("Steps"=w315:T22)
        n156 = Insert Into Array(array=w315, index=w301, new element=w305) -> (w312:T22)
        n157 = Bundle By Name(cluster=w314, "Steps"=w312) -> (w313:T21)
        n158 = call "BuildStepListFromSteps.vi"("Steps"=w312, "Control Channels"=w306, "Feedback Channels"=w307, "AI"=w308) -> ("Step List"=w303:string[])  [unwired: 11 in]
        n159 = Replace Array Subset(array=w309, new element=w313, index=w300) -> (w304:T4)
        n160 = property on="Program step" class="LstBox (strict)"("Key Focus"=TRUE, "Value"=w301, "Item Names"=w303) -> ()  [unwired: 2 in, 2 out]
      }
      event Value Change {
        n161 = event-data() -> ()  [unwired: 1 in, 1 out]
        n162 = property on="Feature List" class="MCListbox (strict)"() -> ("Value"=w338:i32)  [unwired: 2 in, 2 out]
        n163 = property on="Program step" class="LstBox (strict)"() -> ("Value"=w337:i32)  [unwired: 2 in, 2 out]
        n164 = Select(t="STM", s="Motor", f="N") -> (s? t:f=w349:string)
        n165 = call "STM-program.vi"() -> ("OutDir"=w348:i32, "Out Speed"=w346:i32, "Out Degree"=w347:dbl, "Channels (A:B:C:D...) (Out)"=w326:string)  [unwired: 7 in, 1 out]
        n166 = Increment(x=w337) -> (x+1=w332:i32)
        n167 = Bundle By Name(cluster=w344, "Channel Type"=w349, "Channels"=w326, "Wait/Poll (ms)"=u32 0, "Parameter"=u8 0, "STM-Degree"=w347, "STM-Speed"=w346, "Direction"=w348) -> (w329:T20)
        n168 = Index Array(array=w339, index=w338) -> (element=w342:T21)
        n169 = Unbundle By Name(w342) -> ("Steps"=w343:T22)
        n170 = Insert Into Array(array=w343, index=w332, new element=w329) -> (w340:T22)
        n171 = Bundle By Name(cluster=w342, "Steps"=w340) -> (w341:T21)
        n172 = local write "Motor"(FALSE ("Motor")) -> ()
        n173 = call "BuildStepListFromSteps.vi"("Steps"=w340, "Control Channels"=w336, "Feedback Channels"=w335, "AI"=w334) -> ("Step List"=w330:string[])  [unwired: 11 in]
        n174 = Replace Array Subset(array=w339, new element=w341, index=w338) -> (w331:T4)
        n175 = property on="Program step" class="LstBox (strict)"("Key Focus"=TRUE, "Value"=w332, "Item Names"=w330) -> ()  [unwired: 2 in, 2 out]
      }
      event Value Change {
        n176 = event-data() -> ()  [unwired: 1 in, 1 out]
        n177 = property on="Feature List" class="MCListbox (strict)"() -> ("Value"=w352:i32)  [unwired: 2 in, 2 out]
        n178 = Index Array(array=w360, index=w352) -> (element=w363:T21)
        n179 = Bundle By Name(cluster=w369, "Channel Type"="N", "Wait/Poll (ms)"="Wait Time") -> (w365:T20)
        n180 = Unbundle By Name(w363) -> ("Steps"=w364:T22)
        n181 = property on="Program step" class="LstBox (strict)"() -> ("Value"=w366:i32)  [unwired: 2 in, 2 out]
        n182 = Increment(x=w366) -> (x+1=w353:i32)
        n183 = Insert Into Array(array=w364, index=w353, new element=w365) -> (w361:T22)
        n184 = Bundle By Name(cluster=w363, "Steps"=w361) -> (w362:T21)
        n185 = call "BuildStepListFromSteps.vi"("Steps"=w361, "Control Channels"=w358, "Feedback Channels"=w357, "AI"=w355) -> ("Step List"=w356:string[])  [unwired: 11 in]
        n186 = property on="Program step" class="LstBox (strict)"("Item Names"=w356, "Value"=w353, "Key Focus"=TRUE) -> ()  [unwired: 2 in, 2 out]
        n187 = Replace Array Subset(array=w360, new element=w362, index=w352) -> (w359:T4)
      }
      event Value Change {
        n188 = event-data() -> ()  [unwired: 1 in, 2 out]
        n189 = property on="Feature List" class="MCListbox (strict)"() -> ("Value"=w371:i32)  [unwired: 2 in, 2 out]
        n190 = Index Array(array=w382, index=w371) -> (element=w388:T21)
        n191 = property on="Program step" class="LstBox (strict)"() -> ("Value"=w370:i32)  [unwired: 2 in, 2 out]
        n192 = Unbundle By Name(w388) -> ("Item Name"=w386:string, "Item Status"=w385:bool, "Steps"=w384:T22)
        n193 = Equal?(x=w370, y=-1) -> (x = y?=w374:bool)
        n194 = Select(t=0 ("y"), s=w374, f=w370) -> (s? t:f=w372:i32)
        n195 = Delete From Array(array=w384, length=1, index=w372) -> (array with subset deleted=w380:T22)  [unwired: 1 out]
        n196 = Bundle("Item Name"=w386, "Item Status"=w385, "Steps"=w380) -> (w383:T21)  [unwired: 1 in]
        n197 = call "BuildStepListFromSteps.vi"("Steps"=w380, "Control Channels"=w378, "Feedback Channels"=w377) -> ("Step List"=w376:string[])  [unwired: 12 in]
        n198 = Replace Array Subset(array=w382, new element=w383, index=w371) -> (w381:T4)
        n199 = property on="Program step" class="LstBox (strict)"("Item Names"=w376, "Value"=w372, "Key Focus"=TRUE) -> ()  [unwired: 2 in, 2 out]
      }
      event Value Change {
        n200 = event-data() -> ()  [unwired: 1 in, 1 out]
        n201 = for {
          tunnel: w391 -> [w438] mode=indexing
          tunnel: [w433] -> w399 mode=indexing
          shift-right: [w432] -> w400
          shift-left: w407 -> [w435]
          n202 = Unbundle By Name(w438) -> ("Steps"=w439:T22, "Item Name"=w437:string, "Item Status"=w436:bool)
          n203 = Array Size(array=w439) -> (size(s)=w434:i32)
          n204 = case shown="Default" w434 {
            tunnel: w439 -> [_ w446]
            tunnel: w437 -> [_ w448]
            tunnel: w436 -> [_ w447]
            tunnel: [w441 w444] -> w432
            tunnel: w435 -> [w441 w442]
            tunnel: [FALSE TRUE] -> w433
            frame 0 {
            }
            frame Default {
              n205 = Bundle("Item Name"=w448, "Item Status"=w447, "Steps"=w446) -> (w443:T21)  [unwired: 1 in]
              n206 = Build Array (concatenate)(w442, w443) -> (w444:T4)
            }
          }
        }
        n207 = And Array Elements(Boolean array=w399) -> (logical AND=w398:bool)
        n208 = case shown="True" w398 {
          tunnel: [w411 w413] -> w393
          tunnel: w392 -> [_ w421]
          tunnel: [_ w419] -> w401
          tunnel: w400 -> [_ w414]
          tunnel: enum16{"Read", "Write"}."Write" ("Read/Write") -> [_ w420]
          tunnel: "Feature List successfully saved." -> [_ w418]
          tunnel: "Error in saving Feature List." -> [_ w417]
          tunnel: "Can't save Feature List as at least one feature doesn't have steps.\nPlease check." ("message") -> [w412 w416]
          tunnel: w391 -> [w411 _]
          frame False {
            n209 = One Button Dialog(message=w412) -> ()  [unwired: 1 in, 1 out]
          }
          frame True {
            n210 = call "FileIO-ReadWrite-FeatureList.vi"("Filepath"=w421, "Feature List (In)"=w414, "Read/Write"=w420) -> ("Feature List (Out)"=w413:T4, "Error Out"=w419:errorcluster)  [unwired: 11 in]
            n211 = case shown="Error" w419 {
              tunnel: w418 -> [w422 _]
              tunnel: w417 -> [_ w423]
              tunnel: w416 -> [_ _]
              tunnel: [w422 w423] -> w415
              frame No Error {
              }
              frame Error {
              }
            }
            n212 = One Button Dialog(message=w415) -> ()  [unwired: 1 in, 1 out]
          }
        }
        n213 = disable-structure shown="Enabled" {
          frame Disabled {
            n214 = call "Program seq path.vi"() -> ()  [unwired: 11 in, 1 out]
          }
          frame Enabled {
          }
        }
        n215 = Index Array(array=w393, index=0) -> (element=w405:T21)
        n216 = Unbundle By Name(w405) -> ("Steps"=w404:T22)
        n217 = for {
          tunnel: [w430] -> w390 mode=indexing
          tunnel: w393 -> [w425] mode=indexing
          tunnel: [w424] -> _
          i -> [w424]
          n218 = Unbundle By Name(w425) -> ("Item Name"=w431:string, "Item Status"=w429:bool)
          n219 = Select(t="Active", s=w429, f="Inactive") -> (s? t:f=w426:string)
          n220 = Build Array(w431, w426) -> (w430:string[])
        }
        n221 = call "BuildStepListFromSteps.vi"("Steps"=w404, "Control Channels"=w410, "Feedback Channels"=w409, "AI"=w402) -> ("Step List"=w408:string[])  [unwired: 11 in]
        n222 = property on="Program step" class="LstBox (strict)"("Item Names"=w408, "Value"=0 ("Step feautre list")) -> ()  [unwired: 2 in, 2 out]
        n223 = property on="Feature List" class="MCListbox (strict)"("ItemNames"=w390, "Value"=0 ("Feautre list")) -> ()  [unwired: 2 in, 2 out]
      }
      event Value Change {
        n224 = event-data() -> ()  [unwired: 1 in, 1 out]
      }
      event "Program step": Double Click {
        n225 = event-data() -> ("Row"=w465:i32)  [unwired: 1 in, 8 out]
        n226 = property on="Program step" class="LstBox (strict)"() -> ("Item Names"=w466:string[])  [unwired: 2 in, 2 out]
        n227 = Index Array(array=w466, index=w465) -> (element=w456:string)
        n228 = String Length(string=w456) -> (length=w455:i32)
        n229 = String Subset(string=w456, length (rest)=2 ("length (rest)")) -> (substring=w461:string)  [unwired: 1 in]
        n230 = String Subset(string=w456, length (rest)=4 ("length (rest)")) -> (substring=w459:string)  [unwired: 1 in]
        n231 = Less Or Equal?(x=w455, y=0) -> (x <= y?=w452:bool)
        "x <= y?" <- w452
        n232 = Equal?(x=w459, y="Wait") -> (x = y?=w457:bool)
        n233 = Equal?(x=w461, y="Ch") -> (x = y?=w462:bool)
        n234 = case shown="False" w452 {
          tunnel: w474 -> [w485 _]
          tunnel: w473 -> [w484 w548]
          tunnel: w472 -> [w483 _]
          tunnel: w471 -> [w482 _]
          tunnel: w470 -> [w481 _]
          tunnel: [w480 w548] -> w469
          tunnel: [w479 w549] -> w468
          tunnel: w467 -> [w478 w549]
          tunnel: w462 -> [w477 _]
          tunnel: w457 -> [w476 _]
          tunnel: enum32{"Output", "Input"}."Output" ("y") -> [w475 _]
          frame False {
            n235 = case shown="False" w476 {
              tunnel: w485 -> [w502 w535]
              tunnel: w484 -> [w501 w534]
              tunnel: w483 -> [w500 w538]
              tunnel: w482 -> [w499 w537]
              tunnel: w481 -> [w498 w536]
              tunnel: [w497 w533] -> w480
              tunnel: [w496 w532] -> w479
              tunnel: w478 -> [w490 _]
              tunnel: w477 -> [w489 _]
              tunnel: w475 -> [w487 _]
              frame False {
                n236 = call "DO Control.vi"("s"=w489) -> ("Feedback"=w492:i32[], "Parameter (Out)"=w493:u8, "Control Channel"=w495:i32[], "Poll Time (Out)"=w494:u32, "Tab Control 2"=w486:enum32{"Output", "Input"}, "Cancel"=w488:bool)  [unwired: 5 in]
                n237 = Equal?(x=w486, y=w487) -> (x = y?=w491:bool)
                n238 = case shown="False" w488 {
                  tunnel: w502 -> [w527 _]
                  tunnel: w501 -> [w526 w529]
                  tunnel: w500 -> [w525 _]
                  tunnel: w499 -> [w524 _]
                  tunnel: w498 -> [w523 _]
                  tunnel: [w522 w529] -> w497
                  tunnel: [w521 w530] -> w496
                  tunnel: w495 -> [w512 _]
                  tunnel: w494 -> [w511 _]
                  tunnel: w493 -> [w510 _]
                  tunnel: w492 -> [w509 _]
                  tunnel: w491 -> [w503 _]
                  tunnel: w490 -> [_ w530]
                  frame False {
                    n239 = property on="Feature List" class="MCListbox (strict)"() -> ("Value"=w513:i32)  [unwired: 2 in, 2 out]
                    n240 = Index Array(array=w526, index=w513) -> (element=w518:T21)
                    n241 = Select(t="C", s=w503, f="F") -> (s? t:f=w506:string)
                    n242 = Select(t=w512, s=w503, f=w509) -> (s? t:f=w505:i32[])
                    n243 = disable-structure shown="Disabled" {
                      disable-tunnel: w503 -> [w528 _]
                      frame Disabled {
                        n244 = call "Configuration-PromptForChannelParameters_timer.vi"("Control/Feedback\n(Default: False = Feedback)"=w528) -> ()  [unwired: 13 in, 2 out]
                      }
                      frame Enabled {
                      }
                    }
                    n245 = call "ConvertNumericChannelsToStringChannels.vi"("Channels (In)"=w505) -> ("Channels (A:B:C:D...) (Out)"=w504:string)  [unwired: 14 in]
                    n246 = Unbundle By Name(w518) -> ("Steps"=w520:T22)
                    n247 = Bundle By Name(cluster=w527, "Channel Type"=w506, "Channels"=w504, "Wait/Poll (ms)"=w511, "Parameter"=w510) -> (w519:T20)
                    n248 = property on="Program step" class="LstBox (strict)"() -> ("Value"=w514:i32)  [unwired: 2 in, 2 out]
                    n249 = Replace Array Subset(array=w520, new element=w519, index=w514) -> (w516:T22)
                    n250 = Bundle By Name(cluster=w518, "Steps"=w516) -> (w517:T21)
                    n251 = call "BuildStepListFromSteps.vi"("Steps"=w516, "Control Channels"=w523, "Feedback Channels"=w524, "AI"=w525) -> ("Step List"=w521:string[])  [unwired: 11 in]
                    "Step List 2" <- w521
                    n252 = Replace Array Subset(array=w526, new element=w517, index=w513) -> (w522:T4)
                    n253 = property on="Program step" class="LstBox (strict)"("Key Focus"=TRUE, "Value"=w514, "Item Names"=w521) -> ()  [unwired: 2 in, 2 out]
                  }
                  frame True {
                  }
                }
              }
              frame True {
                n254 = property on="Feature List" class="MCListbox (strict)"() -> ("Value"=w539:i32)  [unwired: 2 in, 2 out]
                n255 = call "Timer.vi"() -> ("Wait Time out"=w531:u32)  [unwired: 10 in, 1 out]
                n256 = Index Array(array=w534, index=w539) -> (element=w543:T21)
                n257 = Bundle By Name(cluster=w535, "Channel Type"="N", "Wait/Poll (ms)"=w531) -> (w545:T20)
                n258 = Unbundle By Name(w543) -> ("Steps"=w544:T22)
                n259 = property on="Program step" class="LstBox (strict)"() -> ("Value"=w546:i32)  [unwired: 2 in, 2 out]
                n260 = Replace Array Subset(array=w544, new element=w545, index=w546) -> (w541:T22)
                n261 = Bundle By Name(cluster=w543, "Steps"=w541) -> (w542:T21)
                n262 = call "BuildStepListFromSteps.vi"("Steps"=w541, "Control Channels"=w536, "Feedback Channels"=w537, "AI"=w538) -> ("Step List"=w532:string[])  [unwired: 11 in]
                n263 = property on="Program step" class="LstBox (strict)"("Item Names"=w532, "Value"=w546, "Key Focus"=TRUE) -> ()  [unwired: 2 in, 2 out]
                n264 = Replace Array Subset(array=w534, new element=w542, index=w539) -> (w533:T4)
              }
            }
          }
          frame True {
          }
        }
      }
      event Panel Close? {
        n265 = event-data() -> ()  [unwired: 1 in, 1 out]
        n266 = event-data("Discard?"=TRUE) -> ()  [unwired: 1 in, 1 out]
      }
    }
  }
  "Error Out" <- w23
